vi "Example.vi"() -> ()   [LabVIEW 2014]
uses:
  XMSChart/XMSChart.xctl
panel:
  out "XMSChart":cluster{"X":string, "Y":dbl}[](xcontrol)
  in  "Boolean":bool
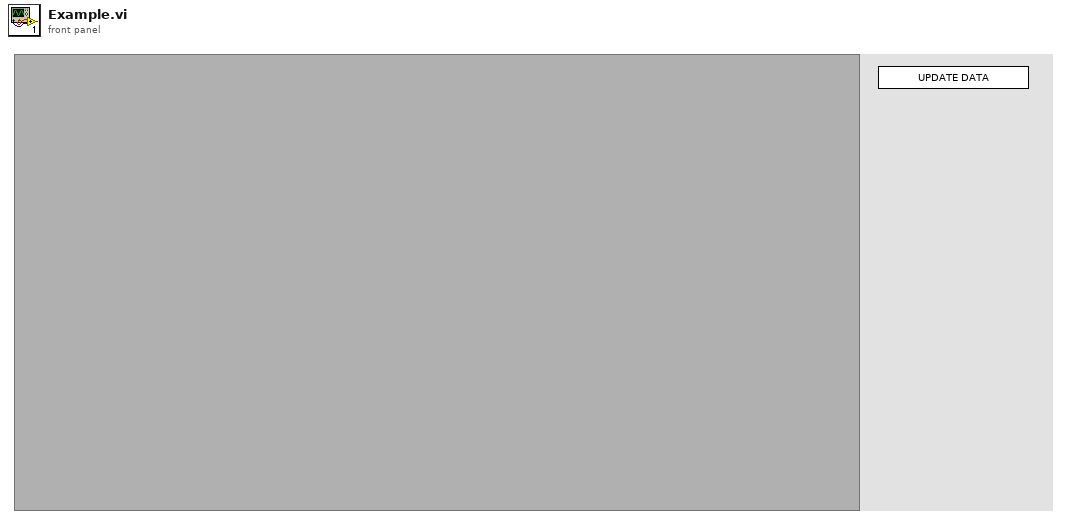
[diagram p1: front panel]
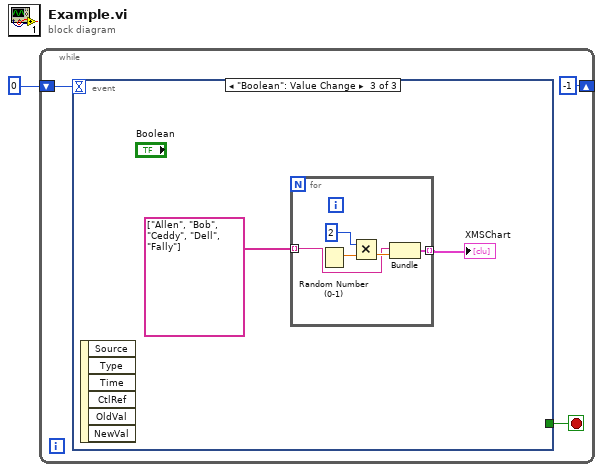
[diagram p0: block diagram]
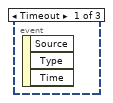
[diagram p2: hidden frame]
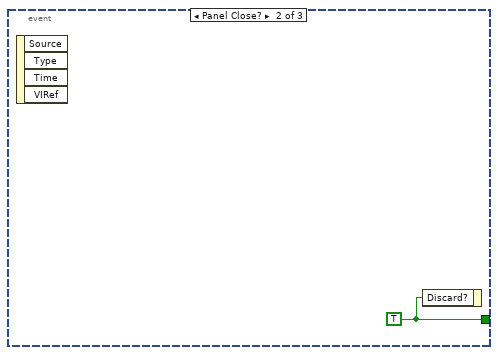
[diagram p3: hidden frame]
diagram:
  n1 = while {
    shift-right: [-1] -> _
    shift-left: 0 -> [w3]
    stop <- w4 stop-if-true
    n2 = event shown="[2] \"Boolean\": Value Change" {
      selector: _ -> [_ _ _]
      dyn-events: _ -> [_ _ _]
      timeout: w3 -> [_ _ _]
      tunnel: [_ w5 _] -> w4
      event Timeout {
        n3 = event-data() -> ()  [unwired: 1 in, 3 out]
      }
      event Panel Close? {
        w5 = TRUE
        n4 = event-data() -> ()  [unwired: 1 in, 4 out]
        n5 = event-data("Discard?"=w5) -> ()  [unwired: 1 in, 1 out]
      }
      event "Boolean": Value Change {
        n6 = event-data() -> ()  [unwired: 1 in, 6 out]
        n7 = for {
          tunnel: [w11] -> w7 mode=indexing
          tunnel: string[] ["Allen", "Bob", "Ceddy", "Dell", "Fally"] -> [w8] mode=indexing
          n8 = Random Number (0-1)() -> (number: 0 to 1=w12:dbl)
          n9 = Multiply(x=2, y=w12) -> (x*y=w10:dbl)
          n10 = Bundle(w8, w10) -> (w11:cluster{string, dbl})  [unwired: 1 in]
        }
        "XMSChart" <- w7
      }
    }
  }
